vi "Generate Data.vi"(8 "Error In":errorcluster, 11 "Numeric in":refnum<class "Numeric.lvclass">) -> (0 "Error Out":errorcluster, 3 "Numeric out":refnum<class "Numeric.lvclass">)   [LabVIEW 2020, in "Numeric.lvclass"]
doc: "The method generates random numeric data to be transmitted."
uses:
  Numeric.lvclass
  Display Data.vi
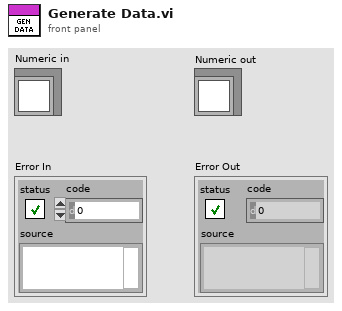
[diagram p1: front panel]
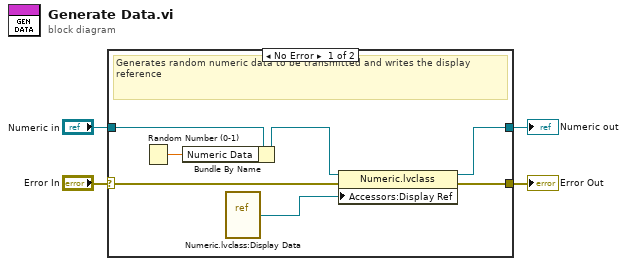
[diagram p0: block diagram]
diagram:
  n1 = case shown="No Error" "Error In" {
    selector: "Error In" -> [w11 w13]
    tunnel: [w8 w13] -> w3
    tunnel: [w6 w12] -> w1
    tunnel: "Numeric in" -> [w10 w12]
    frame No Error {
      # "Generates random numeric data to be transmitted and writes the display reference"
      n2 = Random Number (0-1)() -> (number: 0 to 1=w9:dbl)
      n3 = Bundle By Name(cluster=w10, "Numeric Data"=w9) -> (w7:refnum<class "Numeric.lvclass">)
      n4 = vi-ref "Numeric.lvclass:Display Data.vi"() -> (w5:refnum<vi>)
      n5 = property class="Numeric.lvclass"(reference=w7, error in=w11, "Accessors:Display Ref"=w5) -> (reference out=w6:refnum<class "Numeric.lvclass">, error out=w8:errorcluster)
    }
    frame Error {
    }
  }
  "Error Out" <- w3
  "Numeric out" <- w1
